vi "Array to I32.vi"(1 "DBL Array":cdb[](array[numeric])) -> (0 "I32 Array":i32[](array[numeric]))   [LabVIEW 2018]
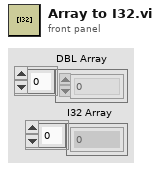
[diagram p1: front panel]
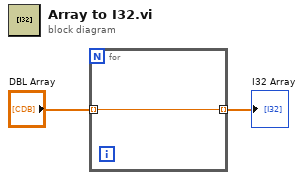
[diagram p0: block diagram]
diagram:
  n1 = for {
    tunnel: "DBL Array" -> [w3] mode=indexing
    tunnel: [w3] -> w1 mode=indexing
  }
  "I32 Array" <- w1
